vi "Run All Caliper Steps.vi"(9 "Analysis_Point_Result":T1[](array[typedef]), 11 "CaliperEntryList":T2[](array[typedef]) {"CaliperType" items=["Distance", "Mid Point", "Perpendicular Projection", "Lines Intersection", "Angle from Horizontal", "Angle from Vertical", "Angle Defined by 3 Points", "Angle Defined by 4 Points", "Bissecting Line", "Mid Line", "Center of Mass", "Area", "Line Fit", "Circle Fit", "Ellipse Fit"]}) -> (3 "CaliperEntryOut":T2[](array[typedef]) {"CaliperType" items=["Distance", "Mid Point", "Perpendicular Projection", "Lines Intersection", "Angle from Horizontal", "Angle from Vertical", "Angle Defined by 3 Points", "Angle Defined by 4 Points", "Bissecting Line", "Mid Line", "Center of Mass", "Area", "Line Fit", "Circle Fit", "Ellipse Fit"]})   [LabVIEW 2019]
uses:
  Controls/CaliperDataEntry.ctl
  Controls/CaliperType.ctl
  Controls/SelectionListEntry.ctl
  Controls/SelectionListEntryPointType.ctl
  Controls/CaliperResult.ctl
  Analysis/Controls/Analysis_Result_To_Caliper.ctl
panel:
  out "error out":errorcluster
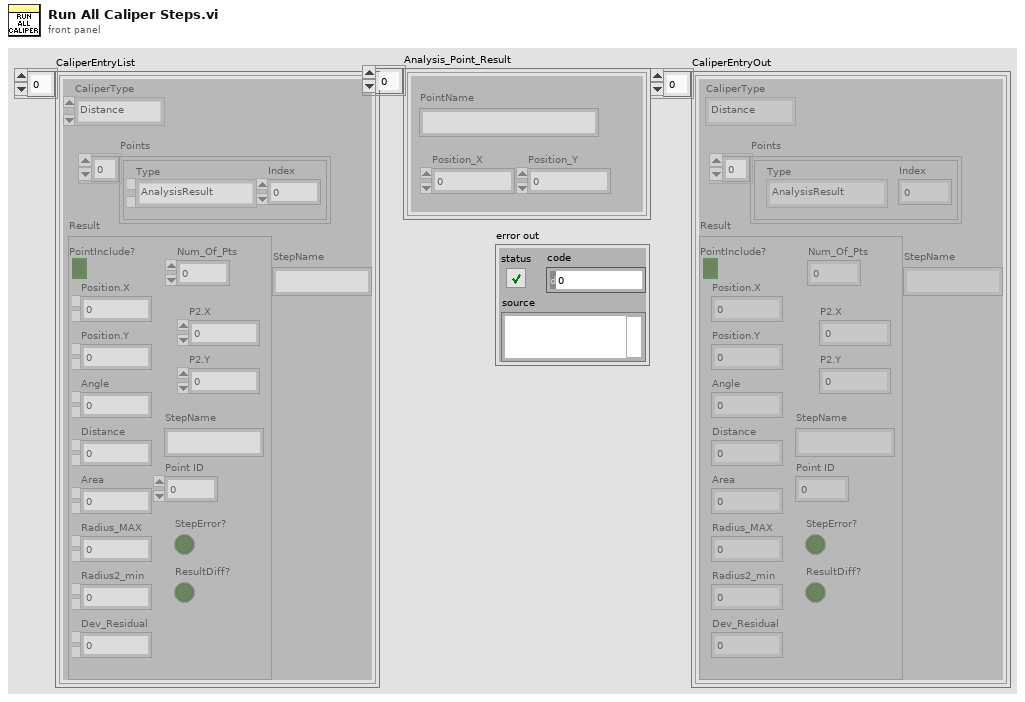
[diagram p1: front panel]
types:
  T1 = typedef "Analysis_Result_To_Caliper.ctl" = cluster{"PointName":string, "Position_X":dbl, "Position_Y":dbl}
  T2 = typedef "CaliperDataEntry.ctl" = cluster{"CaliperType":T3, "Points":T4[], "Result":T6, "StepName":string}
  T3 = typedef "CaliperType.ctl" = u32
  T4 = typedef "SelectionListEntry.ctl" = cluster{"Type":T5, "Index":i32}
  T5 = typedef "SelectionListEntryPointType.ctl" = enum16{"AnalysisResult", "CaliperResult"}
  T6 = typedef "CaliperResult.ctl" = cluster{"PointInclude?":bool, "Num_Of_Pts":u8, "Position.X":dbl, "Position.Y":dbl, "Angle":dbl, "Distance":dbl, "Area":dbl, "Radius_MAX":dbl, "Radius2_min":dbl, "Dev_Residual":dbl, "P2.X":dbl, "P2.Y":dbl, "StepName":string, "Point ID":u8, "StepError?":bool, "ResultDiff?":bool}
  T7 = typedef "CaliperDataEntry_SinglePoint.ctl" = cluster{"CaliperType":T3, "Points":T4[], "Result":T8, "StepName":string}
  T8 = typedef "CaliperResult_SinglePoint.ctl" = cluster{"PointInclude?":bool, "Position.X":dbl, "Position.Y":dbl, "Angle":dbl, "Distance":dbl, "Area":dbl, "Radius_MAX":dbl, "Radius2_min":dbl, "Dev_Residual":dbl, "StepName":string, "Point ID":u8, "StepError?":bool, "ResultDiff?":bool}
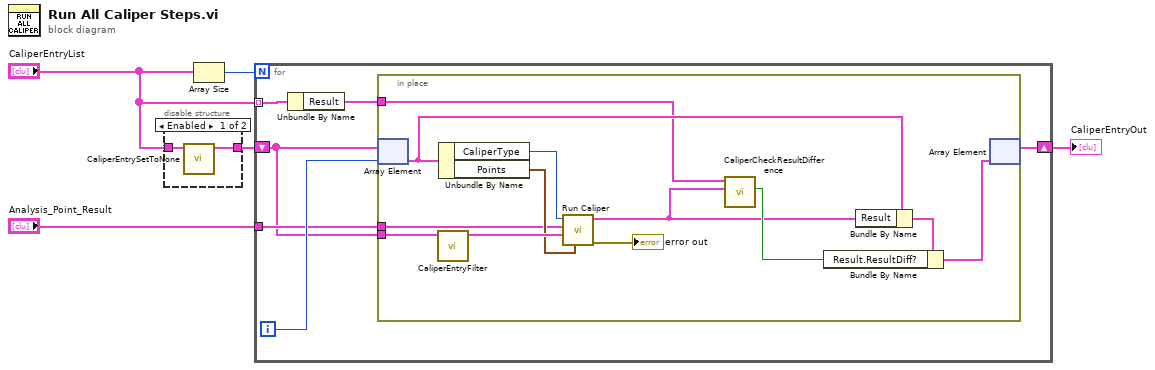
[diagram p0: block diagram]
diagram:
  n1 = disable-structure shown="Enabled" {
    disable-tunnel: [w7 w8] -> w4
    disable-tunnel: "CaliperEntryList" -> [w6 w8]
    frame Enabled {
      n2 = call "CaliperEntrySetToNone.vi"("CaliperEntryList"=w6) -> ("CaliperEntryOut"=w7:T2[])  [unwired: 9 in, 1 out]
    }
    frame Disabled {
    }
  }
  n3 = Array Size(array="CaliperEntryList") -> (size(s)=w5:i32)
  n4 = for {
    N: w5 -> [_]
    tunnel: "Analysis_Point_Result" -> [w13]
    shift-right: [w11] -> w3
    shift-left: w4 -> [w12]
    tunnel: "CaliperEntryList" -> [w10] mode=indexing
    i -> [w14]
    n5 = Unbundle By Name(w10) -> ("Result"=w9:T6)
    n6 = in-place {
      in-place-border: w13 -> [w23]
      in-place-border: w12 -> [w22]
      in-place-border: w9 -> [w15]
      n7 = in-place-array #1(w12, w14) -> (w21:T2)
      n8 = call "CaliperEntryFilter.vi"("CaliperEntryList"=w22) -> ("FilteredCaliperEntry"=w26:T7[])  [unwired: 10 in]
      n9 = Unbundle By Name(w21) -> ("CaliperType"=w25:T3, "Points"=w24:T4[])
      n10 = call "Run Caliper.vi"("SelectionList"=w24, "FilteredCaliperEntry"=w26, "Analysis_Point_Result"=w23, "CaliperType"=w25) -> ("error out"=→"error out":errorcluster, "Result"=w16:T6)  [unwired: 5 in, 1 out]
      n11 = call "CaliperCheckResultDifference.vi"("New Result"=w16, "Old Result"=w15) -> ("ResultDiff?"=w17:bool)  [unwired: 9 in]
      n12 = Bundle By Name(cluster=w21, "Result"=w16) -> (w19:T2)
      n13 = Bundle By Name(cluster=w19, "Result.ResultDiff?"=w17) -> (w18:T2)
      n14 = in-place-array #1(w18) -> (w11:T2[])  [unwired: 1 out]
    }
  }
  "CaliperEntryOut" <- w3
